vi "Motion_Read Gantry Discretes.vi"(8 "error in (no error)":errorcluster, 11 "TCP Connection Refnum in":refnum<k5>) -> (0 "error out":errorcluster, 2 "Gantry Discretes":T1, 3 "TCP Connection Refnum (dup)":refnum<k5>)   [LabVIEW 2010]
uses:
  <vilib>/NI Modbus.llb/MB Ethernet Master Query Read Discrete Inputs (poly).vi
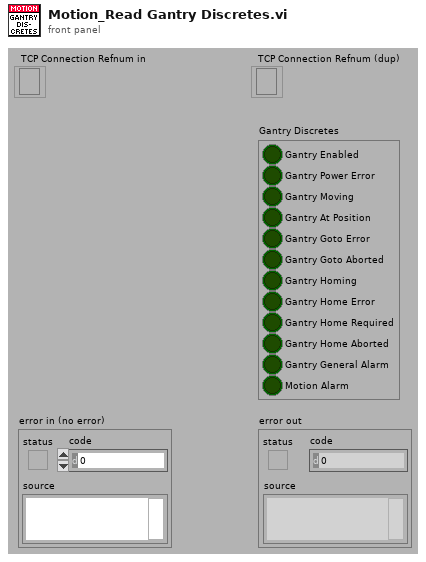
[diagram p1: front panel]
types:
  T1 = cluster{"Gantry Enabled":bool, "Gantry Power Error":bool, "Gantry Moving":bool, "Gantry At Position":bool, "Gantry Goto Error":bool, "Gantry Goto Aborted":bool, "Gantry Homing":bool, "Gantry Home Error":bool, "Gantry Home Required":bool, "Gantry Home Aborted":bool, "Gantry General Alarm":bool, "Motion Alarm":bool}
  T2 = cluster{"[0]":bool, "[1]":bool, "[2]":bool, "[3]":bool, "[4]":bool, "[5]":bool, "[6]":bool, "[7]":bool, "[8]":bool, "[9]":bool, "[10]":bool, "[11]":bool}
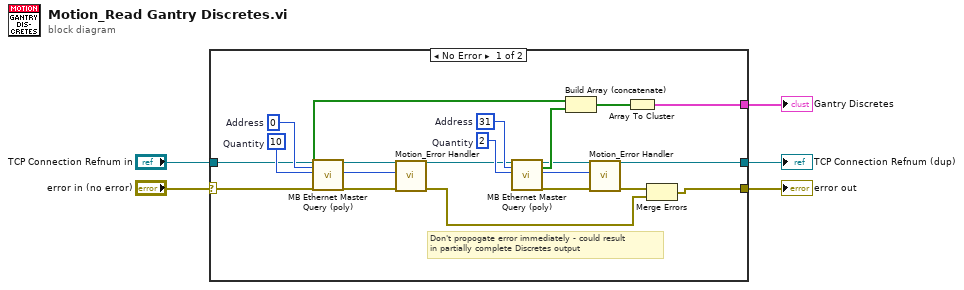
[diagram p0: block diagram]
diagram:
  n1 = case shown="No Error" "error in (no error)" {
    selector: "error in (no error)" -> [w23 w27]
    tunnel: [w24 _] -> w5
    tunnel: [w7 w27] -> w3
    tunnel: [w6 w28] -> w2
    tunnel: "TCP Connection Refnum in" -> [w22 w28]
    frame No Error {
      w18 = u16 2  # Quantity
      w19 = u16 31  # Address
      w25 = u16 10  # Quantity
      w26 = u16 0  # Address
      # "Don't propogate error immediately - could result \nin partially complete Discretes output"
      n2 = call-poly <vilib>:"MB Ethernet Master Query (poly).vi"("TCP Connection Refnum in"=w22, "Starting Address"=w26, "Quantity"=w25, "error in"=w23) -> ("TCP Connection Refnum (dup)"=w15:refnum<k5>, "Discrete Inputs"=w21:bool[], "Exception Code"=w14:u8, "error out"=w16:errorcluster)  [unwired: 12 in]
      n3 = call "Motion_Error Handler.vi"("error in (no error)"=w16, "Exception Code"=w14, "TCP Connection Refnum in"=w15) -> ("error out"=w8:errorcluster, "TCP Connection Refnum (dup)"=w13:refnum<k5>)  [unwired: 7 in]
      n4 = call-poly <vilib>:"MB Ethernet Master Query (poly).vi"("TCP Connection Refnum in"=w13, "Starting Address"=w19, "Quantity"=w18) -> ("TCP Connection Refnum (dup)"=w10:refnum<k5>, "Discrete Inputs"=w17:bool[], "Exception Code"=w12:u8, "error out"=w11:errorcluster)  [unwired: 13 in]
      n5 = Build Array (concatenate)(w21, w17) -> (w20:bool[])
      n6 = call "Motion_Error Handler.vi"("error in (no error)"=w11, "Exception Code"=w12, "TCP Connection Refnum in"=w10) -> ("error out"=w9:errorcluster, "TCP Connection Refnum (dup)"=w6:refnum<k5>)  [unwired: 7 in]
      n7 = Array To Cluster(array=w20) -> (cluster=w24:T2)
      n8 = Merge Errors(w9, w8) -> (w7:errorcluster)
    }
    frame Error {
    }
  }
  "Gantry Discretes" <- w5
  "error out" <- w3
  "TCP Connection Refnum (dup)" <- w2
